vi "ReadyState.vi"(8 "error in (no error)":errorcluster, 10 "Cluster in":T2, 11 "Enum in":T1) -> (0 "error out":errorcluster, 2 "Cluster out":T2, 3 "Enum":T1)   [LabVIEW 2018]
uses:
  Type_Def Actuator Controls.ctl
  Type_Def_ControlState.ctl
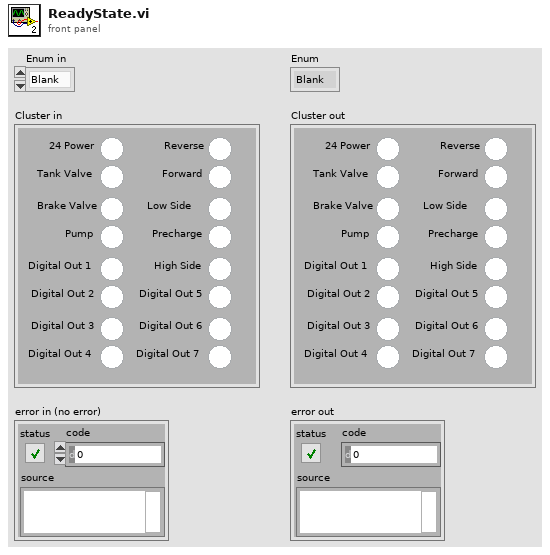
[diagram p1: front panel]
types:
  T1 = typedef "Type_Def_ControlState.ctl" = enum16{"Blank", "Systems Check", "Idle", "Ready", "Pushing", "CrawlingPrecharge", "Braking", "Fault", "Boot Up", "Unpowered", "Crawling", "Shutdown", "Service Push", "Service Wait", "Vent", "Precharge", "Cooldown"}
  T2 = typedef "Type_Def Actuator Controls.ctl" = cluster{"Reverse ":bool, "Forward":bool, "Low Side":bool, "Precharge":bool, "High Side":bool, "Digital Out 5":bool, "Digital Out 6":bool, "Digital Out 7 ":bool, "24 Power":bool, "Tank Valve ":bool, "Brake Valve":bool, "Pump":bool, "Digital Out 1 ":bool, "Digital Out 2":bool, "Digital Out 3":bool, "Digital Out 4 ":bool}
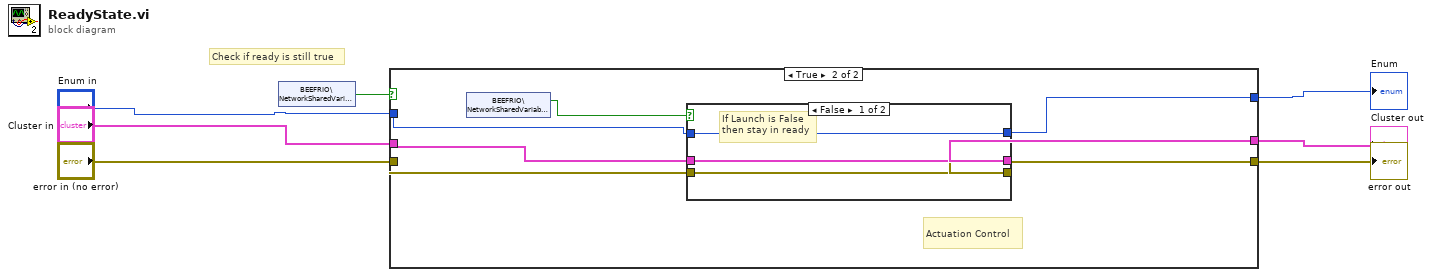
[diagram p0: block diagram]
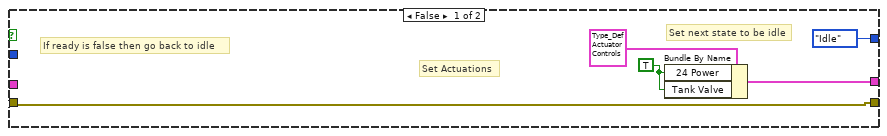
[diagram p2: hidden frame]
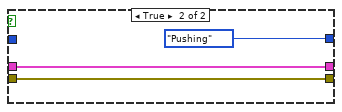
[diagram p3: hidden frame]
diagram:
  # "Check if ready is still true"
  n1 = shared-variable "BEEFRIO\\NetworkSharedVariable.lvlib\\Ready"() -> (w7:bool)  [unwired: 1 in, 1 out]
  n2 = case shown="True" w7 {
    tunnel: "Enum in" -> [_ w19]
    tunnel: [Type_Def_ControlState."Idle" w18] -> w2
    tunnel: "Cluster in" -> [_ w17]
    tunnel: [w9 w16] -> w4
    tunnel: [w8 w15] -> w5
    tunnel: "error in (no error)" -> [w8 w14]
    frame False {
      w11 = TRUE
      # "Set next state to be idle"
      # "Set Actuations"
      # "If ready is false then go back to idle"
      n3 = Bundle By Name(cluster=T2 {"Reverse "=FALSE, "Forward"=FALSE, "Low Side"=FALSE, "Precharge"=FALSE, "High Side"=FALSE, "Digital Out 5"=FALSE, "Digital Out 6"=FALSE, "Digital Out 7 "=FALSE, "24 Power"=FALSE, "Tank Valve "=FALSE, "Brake Valve"=FALSE, "Pump"=FALSE, "Digital Out 1 "=FALSE, "Digital Out 2"=FALSE, "Digital Out 3"=FALSE, "Digital Out 4 "=FALSE}, "24 Power"=w11, "Tank Valve"=w11) -> (w9:T2)
    }
    frame True {
      # "Actuation Control"
      n4 = shared-variable "BEEFRIO\\NetworkSharedVariable.lvlib\\Launch"() -> (w13:bool)  [unwired: 1 in, 1 out]
      n5 = case shown="False" w13 {
        tunnel: w19 -> [w21 _]
        tunnel: [w21 Type_Def_ControlState."Pushing"] -> w18
        tunnel: w17 -> [w20 w23]
        tunnel: [w20 w23] -> w16
        tunnel: [w22 w24] -> w15
        tunnel: w14 -> [w22 w24]
        frame False {
          # "If Launch is False \nthen stay in ready"
        }
        frame True {
        }
      }
    }
  }
  "error out" <- w5
  "Cluster out" <- w4
  "Enum" <- w2
